vi "Configure Pulse Waveform.vi"(5 "Trailing Edge Time (5.0E-9 s)":dbl[unit]=5e-09 format="%#.6g", 6 "Delay (0 s)":dbl[unit], 7 "Leading Edge Time (5.0E-9 s)":dbl[unit]=5e-09 format="%#.6g", 8 "error in (no error)":errorcluster, 9 "Duty Cycle (50%)":dbl=50.0, 10 "Channel (0: Channel 1)":T1 items=["Channel 1", "Channel 2"], 11 "VISA resource name":refnum<visa-resource-name>) -> (0 "error out":errorcluster, 3 "VISA resource name out":refnum<visa-resource-name>)   [LabVIEW 2012, in "Tektronix AFG 3000 Series.lvlib"]
doc: "Configures parameters for pulse waveforms which include channel, leading edge time, trailing edge time, duty cycle, and delay."
uses:
  Tektronix AFG 3000 Series.lvlib
  controls.llb/Channel.ctl
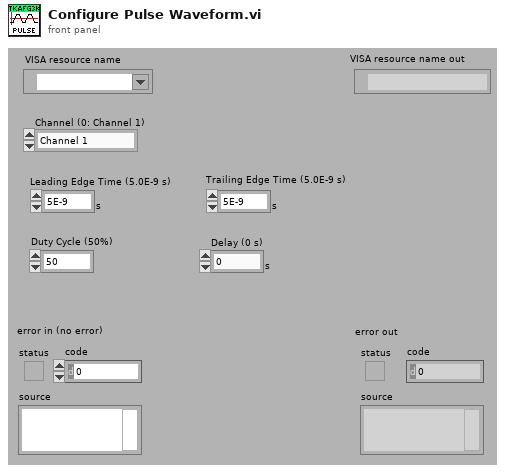
[diagram p1: front panel]
types:
  T1 = typedef "Channel.ctl" = u16
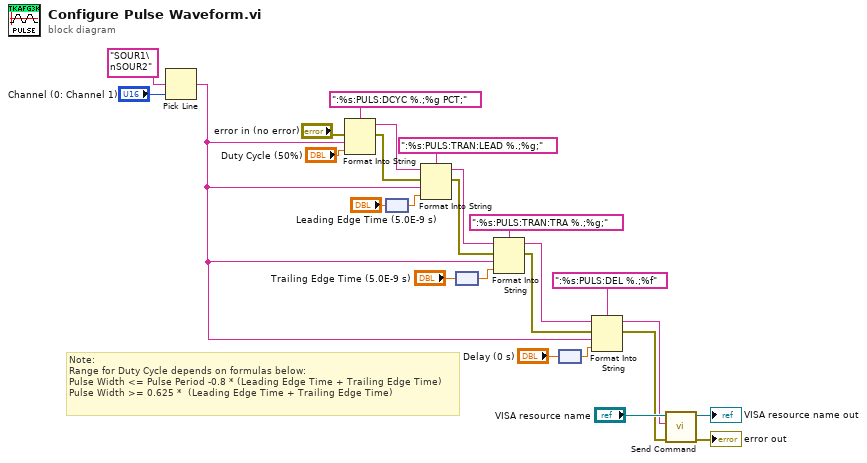
[diagram p0: block diagram]
diagram:
  # "Note:\nRange for Duty Cycle depends on formulas below:\nPulse Width <= Pulse Period -0.8 * (Leading Edge Time + Trailing Edge Time)\nPulse Width >= 0.625 *  (Leading Edge Time + Trailing Edge Time)"
  n1 = Pick Line(multi-line string="SOUR1\nSOUR2" ("string (\"\")"), line index="Channel (0: Channel 1)") -> (output string=w16:string)  [unwired: 1 out]
  n2 = Format Into String(format string=":%s:PULS:DCYC %.;%g PCT;", error in="error in (no error)", w16, "Duty Cycle (50%)") -> (resulting string=w25:string, error out=w14:errorcluster)  [unwired: 1 in]
  n3 = node("Leading Edge Time (5.0E-9 s)") -> (w10:dbl)
  n4 = Format Into String(format string=":%s:PULS:TRAN:LEAD %.;%g;", initial string=w25, error in=w14, w16, w10) -> (resulting string=w24:string, error out=w13:errorcluster)
  n5 = node("Trailing Edge Time (5.0E-9 s)") -> (w8:dbl)
  n6 = Format Into String(format string=":%s:PULS:TRAN:TRA %.;%g;", initial string=w24, error in=w13, w16, w8) -> (resulting string=w17:string, error out=w12:errorcluster)
  n7 = node("Delay (0 s)") -> (w6:dbl)
  n8 = Format Into String(format string=":%s:PULS:DEL %.;%f" ("string"), initial string=w17, error in=w12, w16, w6) -> (resulting string=w3:string, error out=w2:errorcluster)
  n9 = call "Send Command.vi"("error in (no error)"=w2, "write buffer"=w3, "VISA resource name"="VISA resource name") -> ("error out"=→"error out":errorcluster, "VISA resource name out"=→"VISA resource name out":refnum<visa-resource-name>)  [unwired: 7 out]
